vi "Open Connection.vi"(8 "error in (no error)":errorcluster, 9 "Settings file":path, 10 "Connection settings":T1, 11 "Sensor General Class in":refnum<class "Sensor General Class.lvclass">) -> (0 "error out":errorcluster, 3 "Sensor General Class out":refnum<class "Sensor General Class.lvclass">)   [LabVIEW 2020, in "Sensor General Class.lvclass"]
uses:
  Sensor General Class.lvclass
  Connection settings.ctl
  <vilib>/Instr/_visa.llb/VISA Open Access Mode.ctl
  Sensor General Class.lvclass/Sensor General Class.ctl
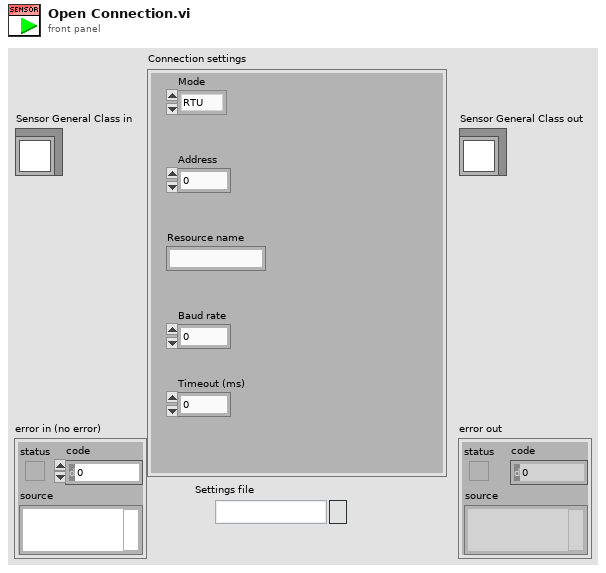
[diagram p1: front panel]
types:
  T1 = typedef "Sensor General Class.lvclass/Connection settings.ctl" = cluster{"Resource name":string, "Baud rate":u16, "Mode":enum16{"RTU", "ASCII"}, "Address":u16, "Timeout (ms)":u16}
  T2 = cluster{"Data registers":cluster{"index":i32, "name":string, "register":u16, "word count":u16}[], "Configuration":cluster{"index":i32, "name":string, "register":u16, "word count":u16, "Write":bool}[]}
  T3 = typedef "VISA Open Access Mode.ctl" = u32
  T4 = cluster{"index":i32, "name":string, "register":u16, "word count":u16}[]
  T5 = cluster{"index":i32, "name":string, "register":u16, "word count":u16, "Write":bool}[]
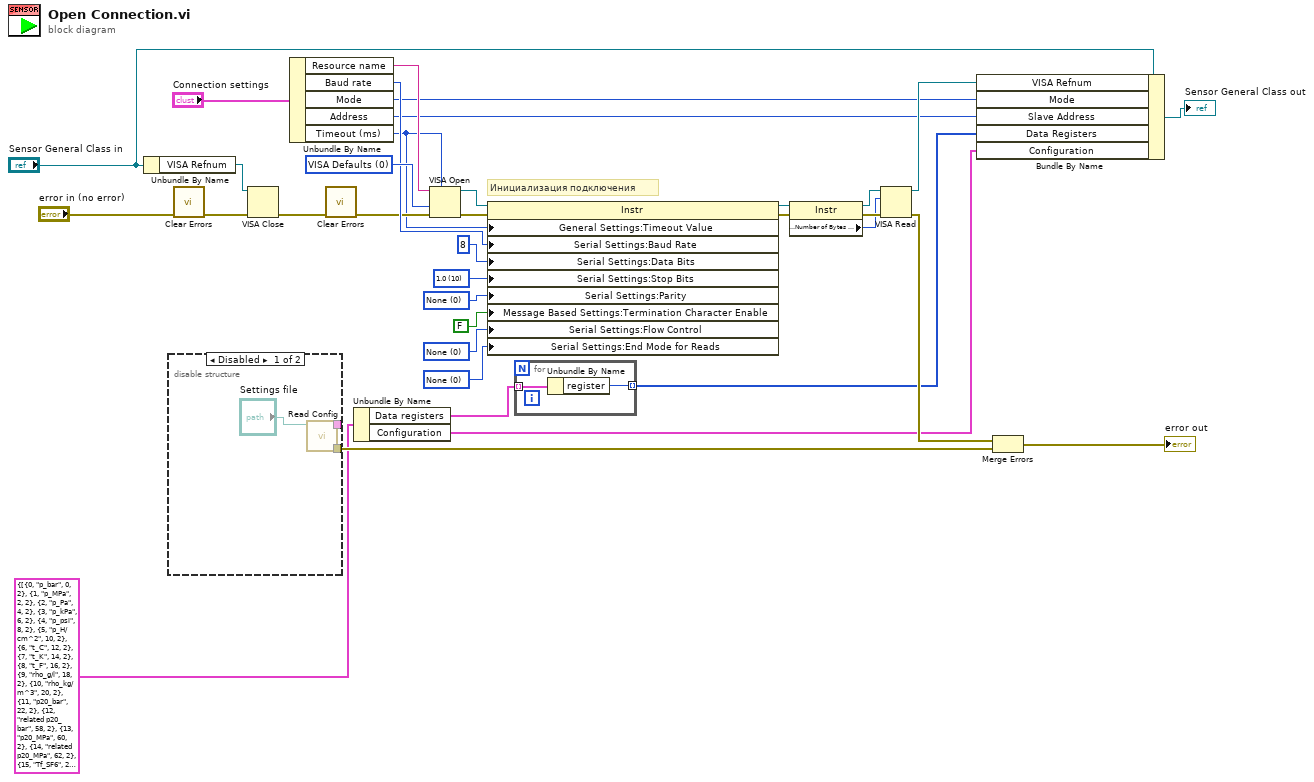
[diagram p0: block diagram]
diagram:
  w22 = T3 0 items=["VISA Defaults"=0, "Exclusive Lock"=1, "Load Configured Settings"=4] ("Access Mode")
  w33 = u16 0 items=["None", "Odd", "Even", "Mark", "Space"] ("Serial Settings:Parity")
  w32 = u16 0 items=["None", "XON/XOFF", "RTS/CTS", "XON/XOFF & RTS/CTS", "DTR/DSR", "XON/XOFF & DTR/DSR"] ("Serial Settings:Flow Control")
  w25 = u16 0 items=["None", "LastBit", "TermChar"] ("Serial Settings:Serial End Mode for Reads")
  w23 = u16 10 items=["1.0"=10, "1.5"=15, "2.0"=20] ("Serial Settings:Serial Stop Bits")
  # "Инициализация подключения"
  n1 = Unbundle By Name("Sensor General Class in") -> ("VISA Refnum"=w16:refnum<visa-resource-name>)
  n2 = disable-structure shown="Disabled" {
    disable-tunnel: [w37 _] -> w6
    disable-tunnel: [w36 _] -> _
    frame Disabled {
      n3 = call "Read Config.vi"("file (use dialog)"="Settings file") -> ("error out"=w37:errorcluster, "Config"=w36:T2)  [unwired: 9 in]
    }
    frame Enabled {
    }
  }
  n4 = call <vilib>:"Clear Errors.vi"("error in (no error)"="error in (no error)") -> ("error out"=w11:errorcluster)  [unwired: 5 in, 1 out]
  n5 = VISA Close(VISA resource name=w16, error in (no error)=w11) -> (error out=w15:errorcluster)
  n6 = Unbundle By Name("Connection settings") -> ("Resource name"=w20:string, "Baud rate"=w18:u16, "Mode"=w10:enum16{"RTU", "ASCII"}, "Address"=w9:u16, "Timeout (ms)"=w8:u16)
  n7 = call <vilib>:"Clear Errors.vi"("error in (no error)"=w15) -> ("error out"=w14:errorcluster)  [unwired: 5 in, 1 out]
  n8 = Unbundle By Name(T2 {"Data registers"=[{"index"=0, "name"="p_bar", "register"=0, "word count"=2}, {"index"=1, "name"="p_MPa", "register"=2, "word count"=2}, {"index"=2, "name"="p_Pa", "register"=4, "word count"=2}, {"index"=3, "name"="p_kPa", "register"=6, "word count"=2}, {"index"=4, "name"="p_psi", "register"=8, "word count"=2}, {"index"=5, "name"="p_H/cm^2", "register"=10, "word count"=2}, {"index"=6, "name"="t_C", "register"=12, "word count"=2}, {"index"=7, "name"="t_K", "register"=14, "word count"=2}, {"index"=8, "name"="t_F", "register"=16, "word count"=2}, {"index"=9, "name"="rho_g/l", "register"=18, "word count"=2}, {"index"=10, "name"="rho_kg/m^3", "register"=20, "word count"=2}, {"index"=11, "name"="p20_bar", "register"=22, "word count"=2}, {"index"=12, "name"="related p20_bar", "register"=58, "word count"=2}, {"index"=13, "name"="p20_MPa", "register"=60, "word count"=2}, {"index"=14, "name"="related p20_MPa", "register"=62, "word count"=2}, {"index"=15, "name"="Tf_SF6", "register"=24, "word count"=2}, {"index"=16, "name"="Td_sf6", "register"=26, "word count"=2}, {"index"=17, "name"="tank Tf_SF6", "register"=28, "word count"=2}, {"index"=18, "name"="tank Td_SF6", "register"=30, "word count"=2}, {"index"=19, "name"="Tf_N2", "register"=32, "word count"=2}, {"index"=20, "name"="Td_N2", "register"=34, "word count"=2}, {"index"=21, "name"="tank Tf_N2", "register"=36, "word count"=2}, {"index"=22, "name"="tank Td_N2", "register"=38, "word count"=2}, {"index"=23, "name"="ppm_v SF6", "register"=40, "word count"=2}, {"index"=24, "name"="ppm_w SF6", "register"=42, "word count"=2}, {"index"=25, "name"="ppm_v N2", "register"=44, "word count"=2}, {"index"=26, "name"="ppm_w N2", "register"=46, "word count"=2}, {"index"=27, "name"="rH", "register"=48, "word count"=2}, {"index"=28, "name"="errors", "register"=200, "word count"=1}], "Configuration"=[{"index"=0, "name"="address", "register"=100, "word count"=1, "Write"=TRUE}, {"index"=1, "name"="baud rate", "register"=101, "word count"=1, "Write"=TRUE}, {"index"=2, "name"="parity check", "register"=102, "word count"=1, "Write"=TRUE}, {"index"=3, "name"="load", "register"=103, "word count"=1, "Write"=TRUE}, {"index"=4, "name"="insulating gas", "register"=130, "word count"=2, "Write"=TRUE}, {"index"=5, "name"="additional component", "register"=105, "word count"=1, "Write"=TRUE}, {"index"=6, "name"="s/n", "register"=106, "word count"=4, "Write"=FALSE}, {"index"=7, "name"="hardware version", "register"=110, "word count"=1, "Write"=FALSE}, {"index"=8, "name"="firmware version", "register"=111, "word count"=1, "Write"=FALSE}, {"index"=9, "name"="humidity enable", "register"=112, "word count"=1, "Write"=FALSE}, {"index"=10, "name"="tag", "register"=113, "word count"=16, "Write"=FALSE}, {"index"=11, "name"="pressure offset", "register"=140, "word count"=1, "Write"=TRUE}, {"index"=12, "name"="humidity offset", "register"=139, "word count"=1, "Write"=TRUE}, {"index"=13, "name"="temperature offset", "register"=138, "word count"=1, "Write"=TRUE}, {"index"=14, "name"="service code", "register"=800, "word count"=1, "Write"=TRUE}]} ("Config")) -> ("Data registers"=w4:T4, "Configuration"=w2:T5)
  n9 = VISA Open(timeout (0)=w8, access mode=w22, error in (no error)=w14, VISA resource name=w20) -> (VISA resource name=w19:refnum<visa-resource-name>, error out=w17:errorcluster)  [unwired: 1 in]
  n10 = property class="Instr"(reference=w19, error in=w17, "General Settings:Timeout Value"=w8, "Serial Settings:Baud Rate"=w18, "Serial Settings:Data Bits"=u16 8 ("data bits"), "Serial Settings:Stop Bits"=w23, "Serial Settings:Parity"=w33, "Message Based Settings:Termination Character Enable"=FALSE, "Serial Settings:Flow Control"=w32, "Serial Settings:End Mode for Reads"=w25) -> (reference out=w27:refnum<visa-resource-name>, error out=w31:errorcluster)
  n11 = for {
    tunnel: w4 -> [w40] mode=indexing
    tunnel: [w39] -> w3 mode=indexing
    n12 = Unbundle By Name(w40) -> ("register"=w39:u16)
  }
  n13 = property class="Instr"(reference=w27, error in=w31) -> (reference out=w30:refnum<visa-resource-name>, error out=w29:errorcluster, "Serial Settings:Number of Bytes at Serial Port"=w28:u32)
  n14 = VISA Read(VISA resource name=w30, byte count=w28, error in (no error)=w29) -> (VISA resource name out=w13:refnum<visa-resource-name>, error out=w7:errorcluster)  [unwired: 2 out]
  n15 = Bundle By Name(cluster="Sensor General Class in", "VISA Refnum"=w13, "Mode"=w10, "Slave Address"=w9, "Data Registers"=w3, "Configuration"=w2) -> (→"Sensor General Class out":refnum<class "Sensor General Class.lvclass">)
  n16 = Merge Errors(w7, w6) -> (→"error out":errorcluster)
